vi "Set Configuration.vi"(8 "error in (no error)":errorcluster, 10 "thread settings":T1, 11 "UDPlog Thread Configuration in":refnum<class "UDPlog Thread Configuration.lvclass">) -> (0 "error out":errorcluster, 3 "UDPlog Thread Configuration out":refnum<class "UDPlog Thread Configuration.lvclass">)   [LabVIEW 2023, in "UDPlog.lvlib" / "UDPlog Thread Configuration.lvclass"]
uses:
  UDPlog Thread Configuration.lvclass
  UDPlog Thread Configuration.lvclass/UDPlog Thread Configuration.ctl
  Thread Settings.ctl
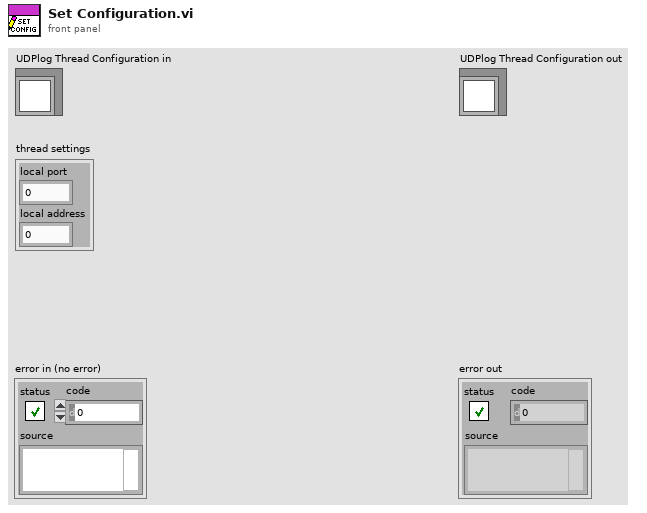
[diagram p1: front panel]
types:
  T1 = typedef "UDPlog.lvlib/UDPlog Thread Configuration.lvclass/Thread Settings.ctl" = cluster{"local port":u16, "local address":u32}
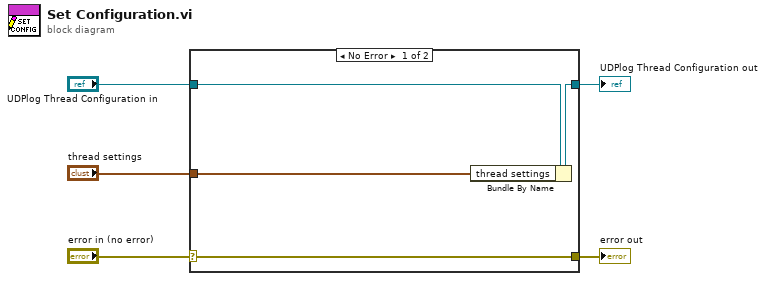
[diagram p0: block diagram]
diagram:
  n1 = case shown="No Error" "error in (no error)" {
    selector: "error in (no error)" -> [w9 w10]
    tunnel: [w9 w10] -> w4
    tunnel: [w7 w11] -> w2
    tunnel: "UDPlog Thread Configuration in" -> [w8 w11]
    tunnel: "thread settings" -> [w6 _]
    frame No Error {
      n2 = Bundle By Name(cluster=w8, "thread settings"=w6) -> (w7:refnum<class "UDPlog Thread Configuration.lvclass">)
    }
    frame Error {
    }
  }
  "error out" <- w4
  "UDPlog Thread Configuration out" <- w2
